vi "ELY (SubVI).vi"(0 "Refnum in":T1, 2 "Leer mas¿?":bool, 5 "Electrolizador":string, 9 "Medidas in":map{string, dbl}(c390), 11 "error in (no error)":errorcluster, 13 "Nodos":string[][](array[string])) -> (1 "Estado":u16, 4 "Refnum out":T1, 6 "Error":u16, 10 "Warning":u16, 12 "Medidas":map{string, dbl}(c390), 14 "StartStop":u16, 15 "error out":errorcluster)   [LabVIEW 2024, in "S7-1200_OPCUA.lvlib"]
uses:
  S7-1200_OPCUA.lvlib
  <vilib>/OPCUA/controls/OPC UA Client Refnum.ctl
  <vilib>/OPCUA/controls/NodeId.ctl
  <vilib>/OPCUA/controls/OPC UA StatusCode.ctl
  <vilib>/OPCUA/client/Multiple Read UInt16.vi
  <vilib>/OPCUA/client/Multiple Read Float.vi
  <vilib>/OPCUA/NI OPC UA Client.lvlib
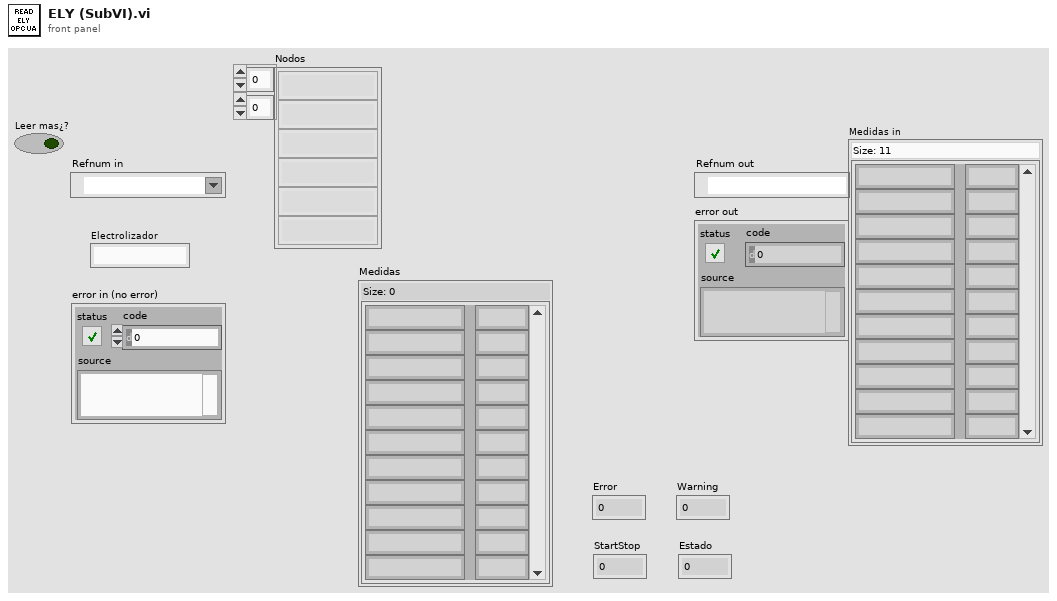
[diagram p1: front panel]
types:
  T1 = typedef "OPC UA Client Refnum.ctl" = refnum<k21>
  T2 = typedef "NodeId.ctl" = string
  T3 = typedef "OPC UA StatusCode.ctl" = u32
  T4 = cluster{"node ID":T2, "value ":u16, "timestamp":timestamp, "status":T3}[]
  T5 = cluster{"node ID":T2, "value ":sgl, "timestamp":timestamp, "status":T3}[]
  T6 = cluster{"node ID":T2, "value ":u16, "timestamp":timestamp, "status":T3}
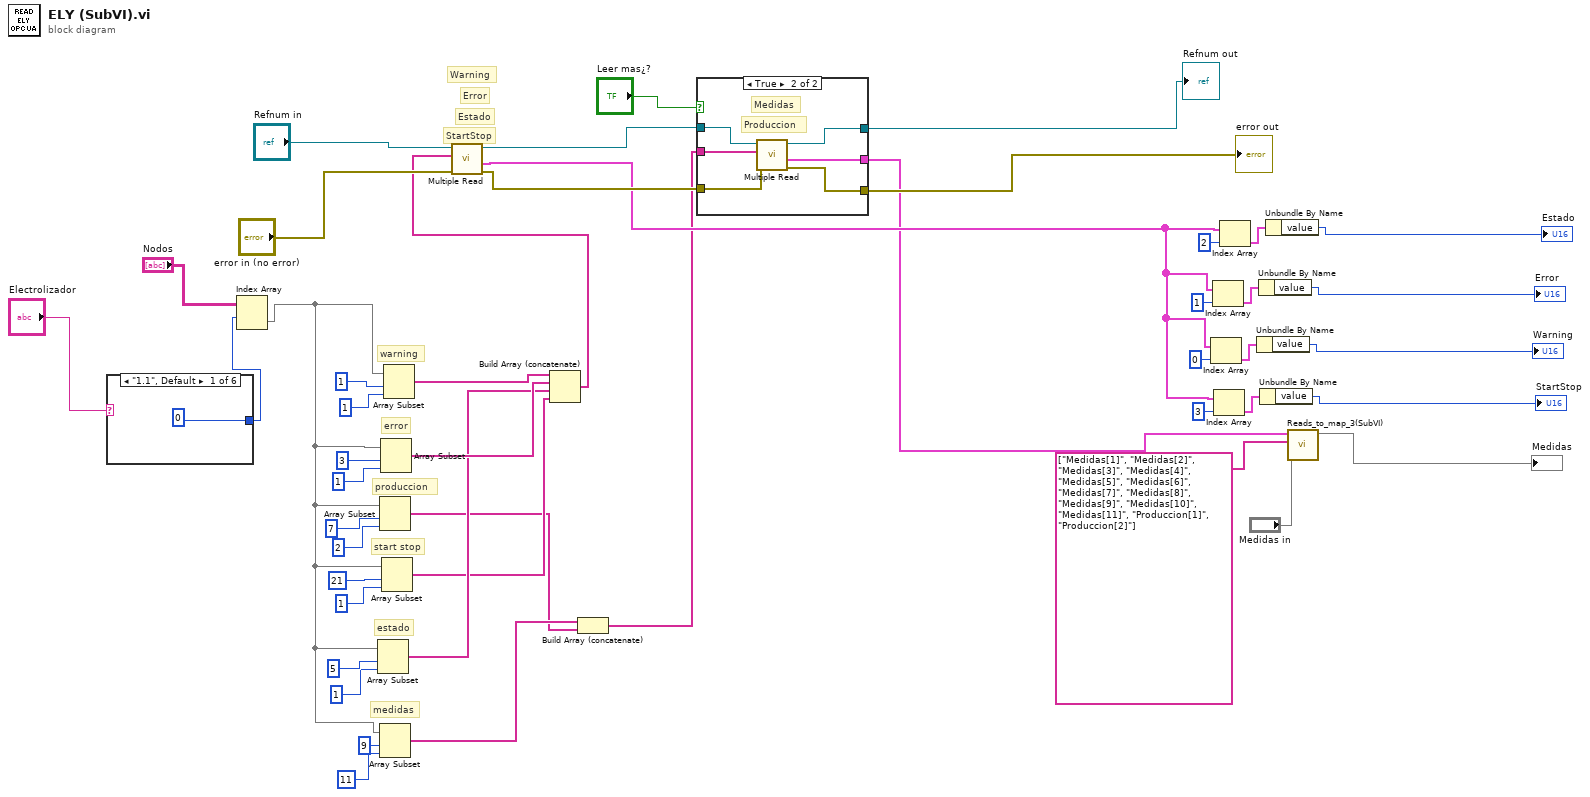
[diagram p0: block diagram]
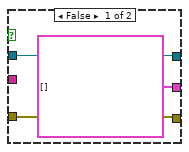
[diagram p2: hidden frame]
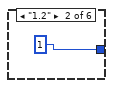
[diagram p3: hidden frame]
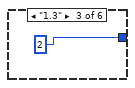
[diagram p4: hidden frame]
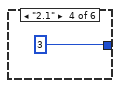
[diagram p5: hidden frame]
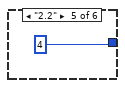
[diagram p6: hidden frame]
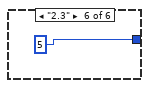
[diagram p7: hidden frame]
diagram:
  # "medidas"
  # "start stop"
  # "estado"
  # "produccion"
  # "warning"
  # "error"
  # "StartStop"
  # "Estado"
  # "Error"
  # "Warning"
  n1 = case shown="\"1.1\", Default" "Electrolizador" {
    tunnel: [0 1 2 3 4 5] -> w5
    frame "1.1", Default {
    }
    frame "1.2" {
    }
    frame "1.3" {
    }
    frame "2.1" {
    }
    frame "2.2" {
    }
    frame "2.3" {
    }
  }
  n2 = Index Array(array="Nodos", index (row)=w5) -> (element=w4:string[])  [unwired: 1 in]
  n3 = Array Subset(array=w4, index=5, length=1) -> (w11:string[])
  n4 = Array Subset(array=w4, index=7, length=2) -> (w8:string[])
  n5 = Array Subset(array=w4, index=9, length=11) -> (w9:string[])
  n6 = Array Subset(array=w4, index=3, length=1) -> (w12:string[])
  n7 = Array Subset(array=w4, index=21, length=1) -> (w10:string[])
  n8 = Array Subset(array=w4, index=1, length=1) -> (w15:string[])
  n9 = Build Array (concatenate)(w15, w12, w11, w10) -> (w37:string[])
  n10 = call-poly <vilib>:"Multiple Read.vi"("error in (no error)"="error in (no error)", "node IDs"=w37, "OPC UA client refnum in"="Refnum in") -> ("error out"=w38:errorcluster, "results"=w36:T4, "OPC UA client refnum out"=w39:T1)  [unwired: 5 in, 1 out]
  n11 = Build Array (concatenate)(w9, w8) -> (w7:string[])
  n12 = case shown="True" "Leer mas¿?" {
    tunnel: w39 -> [w57 w63]
    tunnel: w38 -> [w56 w62]
    tunnel: [w57 w61] -> w35
    tunnel: [w56 w60] -> w34
    tunnel: [T5 [] ("results") w59] -> w1
    tunnel: w7 -> [_ w58]
    frame False {
    }
    frame True {
      # "Produccion"
      # "Medidas"
      n13 = call-poly <vilib>:"Multiple Read.vi"("error in (no error)"=w62, "node IDs"=w58, "OPC UA client refnum in"=w63) -> ("error out"=w60:errorcluster, "results"=w59:T5, "OPC UA client refnum out"=w61:T1)  [unwired: 5 in, 1 out]
    }
  }
  "error out" <- w34
  "Refnum out" <- w35
  n14 = Index Array(array=w36, index=0) -> (element=w31:T6)
  n15 = Index Array(array=w36, index=1) -> (element=w32:T6)
  n16 = Index Array(array=w36, index=3) -> (element=w30:T6)
  n17 = Index Array(array=w36, index=2) -> (element=w33:T6)
  n18 = Unbundle By Name(w31) -> ("value"=→"Warning":u16)
  n19 = Unbundle By Name(w32) -> ("value"=→"Error":u16)
  n20 = Unbundle By Name(w30) -> ("value"=→"StartStop":u16)
  n21 = Unbundle By Name(w33) -> ("value"=→"Estado":u16)
  n22 = call "Reads_to_map_3(SubVI).vi"("Map in"="Medidas in", "Array"=string[] ["Medidas[1]", "Medidas[2]", "Medidas[3]", "Medidas[4]", "Medidas[5]", "Medidas[6]", "Medidas[7]", "Medidas[8]", "Medidas[9]", "Medidas[10]", "Medidas[11]", "Produccion[1]", "Produccion[2]"], "results"=w1) -> ("Map out"=→"Medidas":map{string, dbl})  [unwired: 8 in]
